vi "from string.vi"(8 "error in":errorcluster, 9 "data":string, 10 "version":string, 11 "fixed channel configuration in":refnum<class "AppStateMachine configuration.lvclass">) -> (0 "error out":errorcluster, 3 "fixed channel configuration out":refnum<class "AppStateMachine configuration.lvclass">)   [LabVIEW 2017, in "AppStateMachine configuration.lvclass"]
doc: "Provides an interface for loading a module configuration from a file or other serialized data source. It is recommended that all children of this class store data in two sets--data required for its own initialization, and any data required for parent initialization--and that each implementation uses the <b>Call Parent Method</b> primitive to de-serialize parent information. As a result, it is expected that every module configuration class calls <b>component configuration.lvclass:From String.vi</b>.\nNI Tag Bus Module Framework 1.0.3.43\nNI Systems Engineering"
uses:
  AppStateMachine configuration.lvclass
  AppStateMachine configuration.lvclass/AppStateMachine configuration.ctl
  <vilib>/NI/JSON Support for LabVIEW/JSON Data Classes/JSON Helper/Parsing/Parse Value.vi
  <vilib>/NI/JSON Support for LabVIEW/JSON Data Classes/JSON Helper/To More Specific Type (Object).vi
  <vilib>/NI/JSON Support for LabVIEW/JSON Data Classes/JSON Object/Get Value (Numeric Value).vi
  <vilib>/NI/JSON Support for LabVIEW/JSON Data Classes/JSON Datatype/JSON Null.lvclass
  <vilib>/NI/DCAF/Tag Editor Core/control module/configuration/control module configuration.lvclass
  <vilib>/NI/Configuration Framework/serializable configuration/NISE_CEF_serializable configuration.lvclass
  <vilib>/NI/JSON Support for LabVIEW/JSON Data Classes/JSON Helper/JSON Helper.lvclass
  <vilib>/NI/JSON Support for LabVIEW/JSON Data Classes/JSON Object/JSON Object.lvclass
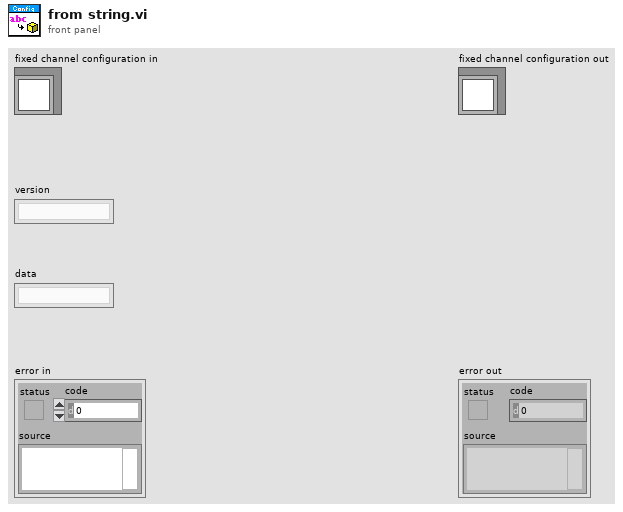
[diagram p1: front panel]
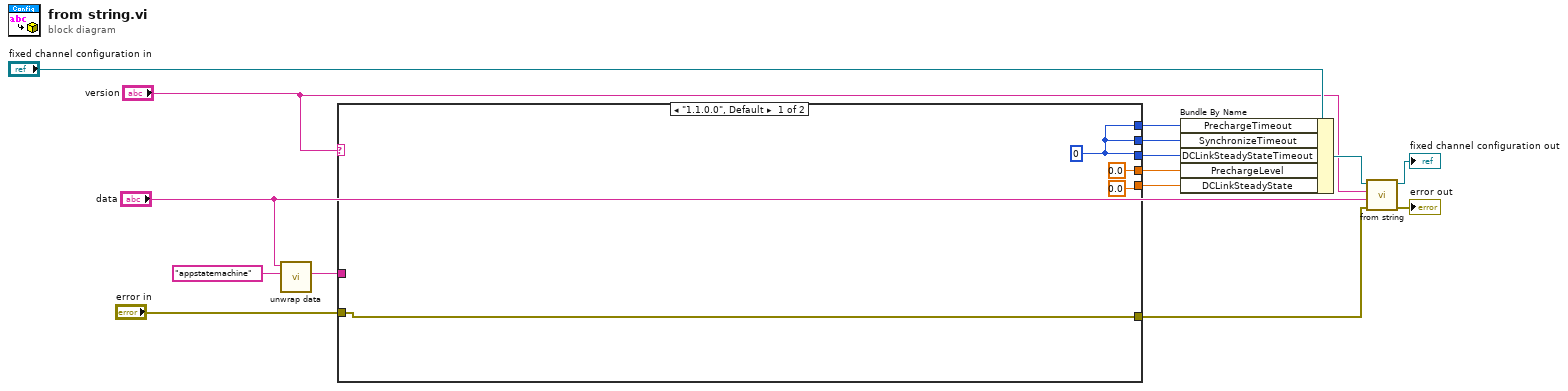
[diagram p0: block diagram]
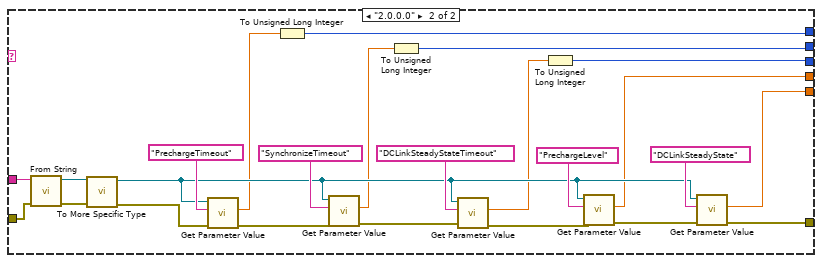
[diagram p2: hidden frame]
diagram:
  n1 = call <vilib>:"unwrap data.vi"("identifier"="appstatemachine", "data to unwrap"="data") -> ("unwrapped data"=w13:string)  [unwired: 8 in, 1 out]
  n2 = case shown="\"1.1.0.0\", Default" "version" {
    tunnel: w13 -> [_ w43]
    tunnel: "error in" -> [w19 w40]
    tunnel: [w19 w29] -> w9
    tunnel: [w16 w24] -> w6
    tunnel: [w16 w22] -> w5
    tunnel: [w16 w20] -> w4
    tunnel: [0.0 ("value") w27] -> w3
    tunnel: [0.0 ("value") w26] -> w2
    frame "1.1.0.0", Default {
      w16 = u32 0
    }
    frame "2.0.0.0" {
      n3 = call <vilib>:"From String.vi"("error in (no error)"=w40, "JSON String"=w43) -> ("error out"=w41:errorcluster, "JSON out"=w42:refnum<class "JSON Null.lvclass">)  [unwired: 8 in]
      n4 = call-poly <vilib>:"To More Specific Type.vi"("error in (no error)"=w41, "JSON Datatype in"=w42) -> ("error out"=w28:errorcluster, "JSON Datatype out"=w34:refnum<class "JSON Object.lvclass">)  [unwired: 8 in]
      n5 = call-poly <vilib>:"Get Parameter Value.vi"("error in (no error)"=w28, "key"="PrechargeTimeout", "JSON Object in"=w34) -> ("error out"=w33:errorcluster, "value"=w25:dbl)  [unwired: 7 in]
      n6 = To Unsigned Long Integer(number=w25) -> (unsigned 32bit integer=w24:u32)
      n7 = call-poly <vilib>:"Get Parameter Value.vi"("error in (no error)"=w33, "key"="SynchronizeTimeout", "JSON Object in"=w34) -> ("error out"=w32:errorcluster, "value"=w23:dbl)  [unwired: 7 in]
      n8 = To Unsigned Long Integer(number=w23) -> (unsigned 32bit integer=w22:u32)
      n9 = call-poly <vilib>:"Get Parameter Value.vi"("error in (no error)"=w32, "key"="DCLinkSteadyStateTimeout", "JSON Object in"=w34) -> ("error out"=w31:errorcluster, "value"=w21:dbl)  [unwired: 7 in]
      n10 = To Unsigned Long Integer(number=w21) -> (unsigned 32bit integer=w20:u32)
      n11 = call-poly <vilib>:"Get Parameter Value.vi"("error in (no error)"=w31, "key"="PrechargeLevel", "JSON Object in"=w34) -> ("error out"=w30:errorcluster, "value"=w27:dbl)  [unwired: 7 in]
      n12 = call-poly <vilib>:"Get Parameter Value.vi"("error in (no error)"=w30, "key"="DCLinkSteadyState", "JSON Object in"=w34) -> ("error out"=w29:errorcluster, "value"=w26:dbl)  [unwired: 7 in]
    }
  }
  n13 = Bundle By Name(cluster="fixed channel configuration in", "PrechargeTimeout"=w6, "SynchronizeTimeout"=w5, "DCLinkSteadyStateTimeout"=w4, "PrechargeLevel"=w3, "DCLinkSteadyState"=w2) -> (w7:refnum<class "AppStateMachine configuration.lvclass">)
  n14 = call-parent <vilib>:"from string.vi"("error in"=w9, "data"="data", "version"="version", "fixed channel configuration in"=w7) -> ("error out"=→"error out":errorcluster, "fixed channel configuration out"=→"fixed channel configuration out":refnum<class "AppStateMachine configuration.lvclass">)  [unwired: 6 in]
